vi "Variant Configuration Error Handler.vi"(7 "Error Code":i32=5801, 8 "error in":errorcluster, 10 "Variant":variant) -> (0 "error out":errorcluster)   [LabVIEW 2018, in "EMS Generic Actor.lvlib" / "EMS Generic.lvclass"]
uses:
  EMS Generic.lvclass
  <vilib>/Utility/Data Type/NI_Data Type.lvlib
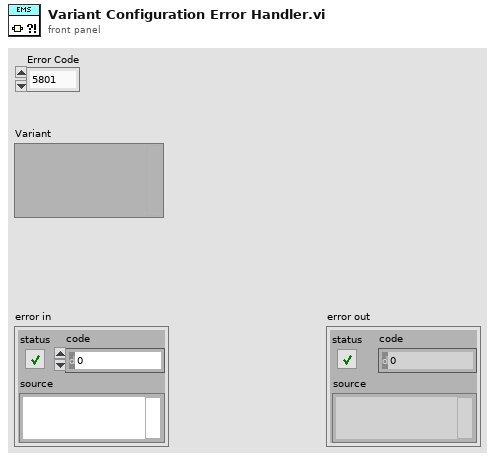
[diagram p1: front panel]
types:
  T1 = typedef "NI_Data Type.lvlib/Data Type.ctl" = enum8{"Invalid Type", "Void", "I8", "I16", "I32", "I64", "U8", "U16", "U32", "U64", "Single Float", "Double Float", "Extended Float", "Single Complex", "Double Complex", "Extended Complex", "Enum U8", "Enum U16", "Enum U32", "Enum U64", "Single Float With Unit", "Double Float With Unit", "Extended Float With Unit", "Single Complex with Unit", "Double Complex with Unit", "Extended Complex with Unit", "Boolean", "String", "Path", "Picture", "Tag", "Array", "Cluster", "Variant", "LV Variant", "Waveform", "Timestamp", "Digital Waveform", "Digital Data", "ExpressData", "Refnum", "External Data", "VI", "Poly VI", "LabVIEW Class Instance", "Fixed Point"}
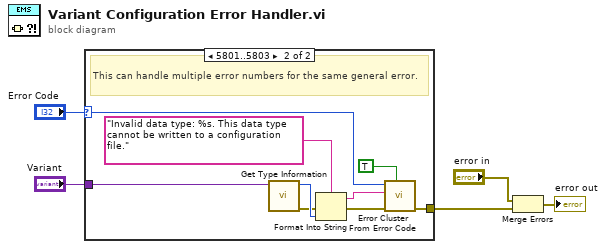
[diagram p0: block diagram]
diagram:
  n1 = case shown="5801..5803" "Error Code" {
    selector: "Error Code" -> [_ w10]
    tunnel: "Variant" -> [_ w9]
    tunnel: [_ w6] -> w2
    frame 0, Default {
    }
    frame 5801..5803 {
      # "This can handle multiple error numbers for the same general error."
      n2 = call <vilib>:"Get Type Information.vi"("Variant"=w9) -> ("error out"=w7:errorcluster, "Type"=w8:T1)  [unwired: 6 in, 3 out]
      n3 = Format Into String(format string="Invalid data type: %s. This data type cannot be written to a configuration file." ("error message (\"\")"), error in=w7, w8) -> (resulting string=w14:string, error out=w13:errorcluster)  [unwired: 1 in]
      n4 = call <vilib>:"Error Cluster From Error Code.vi"("show call chain? (False)"=TRUE, "error in (no error)"=w13, "error message (\"\")"=w14, "error code (0)"=w10) -> ("error out"=w6:errorcluster)  [unwired: 5 in]
    }
  }
  n5 = Merge Errors("error in", w2) -> (→"error out":errorcluster)
